vi "S2C_FORNAX_Poly_DftLogCommand.vi"(8 "Error In":errorcluster, 10 "DftLogCommand":T2={"Partition"="Default", "Message"="DftLogCommand", "M_Command"=0, "M_CommandOptions"=""} {"M_Command" items=["LOG_COMMAND_INVALID", "LOG_COMMAND_CLEAR_ALL", "LOG_COMMAND_CLEAR_EVENT", "LOG_COMMAND_CLEAR_ALARM", "LOG_COMMAND_CLEAR_RFID", "LOG_COMMAND_ROTATE_ALL", "LOG_COMMAND_ROTATE_EVENT", "LOG_COMMAND_ROTATE_ALARM", "LOG_COMMAND_ROTATE_RFID", "LOG_COMMAND_CLEAR_RFDATA", "LOG_COMMAND_RF_DATA_ALL_MODES", "LOG_COMMAND_RF_DATA_LIGASURE_ONLY", "LOG_COMMAND_CLEAR_USAGE", "LOG_COMMAND_ROTATE_USAGE", "NUM_LOG_COMMANDS"]}, 11 "Settings":T3={"Driver"="Fornax", "Command"="DftLogCommand", "Return"="ErrorStatus", "Parameters"="", "Timeout"=10.0}) -> (0 "Error Out":errorcluster, 3 "Response":string)   [LabVIEW 2015]
uses:
  Typedefs/LogCommand.ctl
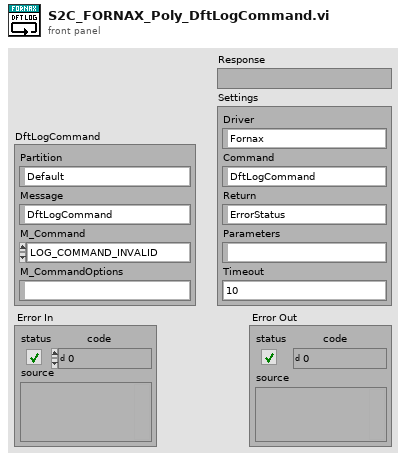
[diagram p1: front panel]
types:
  T1 = typedef "LogCommand.ctl" = i16
  T2 = cluster{"Partition":string, "Message":string, "M_Command":T1, "M_CommandOptions":string}
  T3 = cluster{"Driver":string, "Command":string, "Return":string, "Parameters":string, "Timeout":dbl}
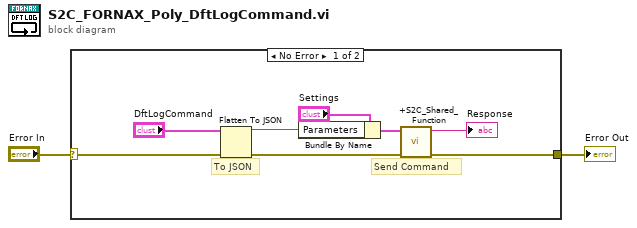
[diagram p0: block diagram]
diagram:
  n1 = case shown="No Error" "Error In" {
    selector: "Error In" -> [w6 w11]
    tunnel: [w5 w11] -> w1
    frame No Error {
      # "To JSON"
      # "Send Command"
      n2 = Flatten To JSON(anything="DftLogCommand", error in (no error)=w6) -> (JSON string=w7:string, 11:w9:errorcluster)  [unwired: 1 in]
      n3 = Bundle By Name(cluster="Settings", "Parameters"=w7) -> (w10:T3)
      n4 = call "+S2C_Shared_Function.vi"("Error In"=w9, "Settings"=w10) -> ("Error Out"=w5:errorcluster, "Response"=→"Response":string)  [unwired: 8 in]
    }
    frame Error {
    }
  }
  "Error Out" <- w1
